vi "Init Device.vi"(7 "Layout Ref":refnum<vi>, 8 "error in (no error)":errorcluster, 10 "Chan# Array":i32[](array[numeric]), 11 "Slave_Line in":refnum<class "Slave_Line.lvclass">) -> (0 "error out":errorcluster, 3 "Slave_Line out":refnum<class "Slave_Line.lvclass">)   [LabVIEW 2013, in "Slave_Line.lvclass"]
doc: "Initialize the correct columns and their default appearance.\nUse the front panel to change default appearance of the device in the Add/Manage devices.\n\nOpen a specific device implementation for details."
uses:
  Slave_Line.lvclass
  TypeDefs/DigitalColumnAppearCluster.ctl
  ColumnVIs/DigitalCol/DigitalCol.lvclass
  Slave_Line.lvclass/Slave_Line.ctl
  ColumnVIs/Column/Column.lvclass
panel:
  in  "Slave Column":T1={"Column Name"="", "Width"=15, "Bkgd"=[1985280, 6618880, 14090026], "Text"=[16448250, 0, 0]}
  # "Open a specific devices override of this VI for implementation."
  # "Intended functionality:\n------------------------\nPlace controls here for Device programmer OR advanced user to configure\ntypical layout in the table.\n\nDisplay Info.vi (called on add/manage device) will be where typical user can fine tune."
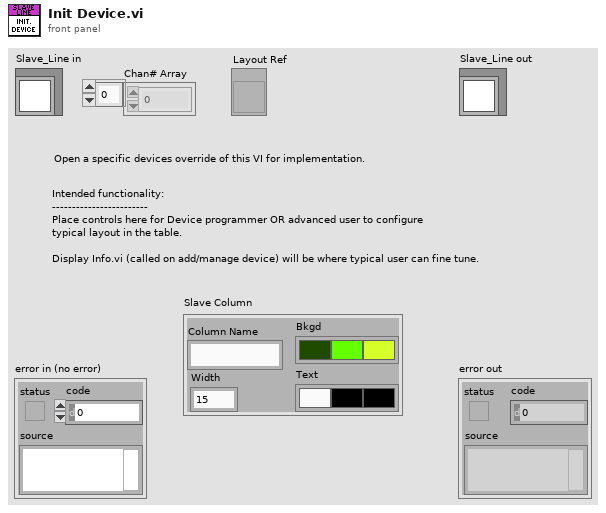
[diagram p1: front panel]
types:
  T1 = typedef "DigitalColumnAppearCluster.ctl" = cluster{"Column Name":string, "Width":u32, "Bkgd":u32[], "Text":u32[]}
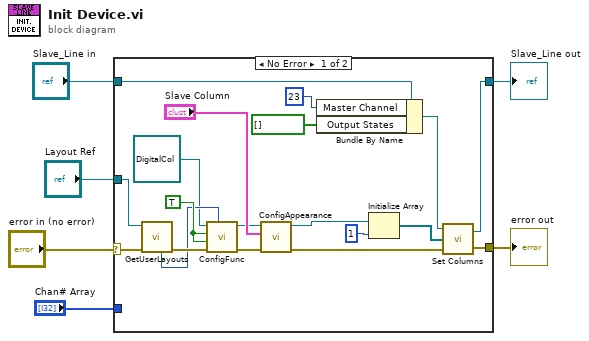
[diagram p0: block diagram]
diagram:
  n1 = case shown="No Error" "error in (no error)" {
    selector: "error in (no error)" -> [w8 w26]
    tunnel: "Chan# Array" -> [_ _]
    tunnel: "Slave_Line in" -> [w7 w27]
    tunnel: [w21 w26] -> w4
    tunnel: [w16 w27] -> w3
    tunnel: "Layout Ref" -> [w12 _]
    frame No Error {
      w15 = TRUE ("Disableable? (True)")
      n2 = call "GetUserLayouts.vi"("error in (no error)"=w8, "Layout Ring Refnum"=w12) -> ("error out"=w14:errorcluster, "Num User Layouts"=w13:i32)  [unwired: 5 in, 3 out]
      n3 = call "ConfigFunc.vi"("Num Layouts (ignored)"=w13, "error in (no error)"=w14, "isVariable? (True)"=w15, "Disableable? (True)"=w15, "Column in"=refnum<class "DigitalCol.lvclass"> refnum ("DigitalCol.lvclass")) -> ("error out"=w11:errorcluster, "Column out"=w9:refnum<class "DigitalCol.lvclass">)  [unwired: 5 in]
      n4 = call "ConfigAppearance.vi"("error in (no error)"=w11, "Column Appearance"="Slave Column", "Column in"=w9) -> ("error out"=w22:errorcluster, "Column out"=w19:refnum<class "DigitalCol.lvclass">)  [unwired: 7 in]
      n5 = Bundle By Name(cluster=w7, "Master Channel"=23, "Output States"=bool[] []) -> (w17:refnum<class "Slave_Line.lvclass">)
      n6 = Initialize Array(w19, 1 ("dimension size")) -> (w18:refnum<class "DigitalCol.lvclass">[])
      n7 = call-dynamic "Set Columns.vi"("error in (no error)"=w22, "Columns"=w18, "Device in"=w17) -> ("error out"=w21:errorcluster, "Device out"=w16:refnum<class "Slave_Line.lvclass">)  [unwired: 1 in]
    }
    frame Error {
    }
  }
  "error out" <- w4
  "Slave_Line out" <- w3
